vi "temp.vi"   [LabVIEW 2017]
uses:
  Configuration/Controls/Config Data.ctl
  Configuration/Controls/Config CMD.ctl
  ATM Controller/Controls/Controller Overhead.ctl
  ATM Controller/Controls/Controller States.ctl
  ATM Controller/Controls/Controller Message Data.ctl
  ATM Controller/Controls/Controller Message Name.ctl
  Views/User Console View/Controls/User Console - Keypad.ctl
  Views/User Console View/Controls/User Console - Transactions.ctl
  ATM Controller/Controls/Controller CMD.ctl
  Views/User Console View/Controls/User Console - Transaction Enum.ctl
  Error Handler/Controls/Error Data.ctl
  Error Handler/Controls/Error Type.ctl
types:
  T1 = typedef "Controller Message Data.ctl" = cluster{"Transaction":string, "Message":string, "Card Read":bool, "Message Name":T2}
  T2 = typedef "Controller Message Name.ctl" = enum16{"Welcome", "Login", "Idle", "Invalid Login", "Terminate", "Deposit", "Withdrawal", "Fast Cash", "Withdrawal Complete", "Withdrawal Failed", "Balance Inquiry"}
  T3 = typedef "User Console - Transaction Enum.ctl" = enum16{"Balance Inquiry", "Deposit", "Withdrawal", "Fat Cash", "New Transaction", "Terminate Session"}
  T4 = typedef "Controller CMD.ctl" = cluster{"Controller State":T5, "Variant":variant}
  T5 = typedef "Controller States.ctl" = enum16{"Idle", "Init", "Display Message", "Login", "Balance Inquiry", "Deposit", "Withdrawal", "Fast Cash", "Terminate"}
  T6 = typedef "User Console - Transactions.ctl" = cluster{"Balance Inquiry":bool, "Deposit":bool, "Withdrawal":bool, "Fast Cash":bool, "New Transaction":bool, "Terminate":bool}
  T7 = typedef "User Console - Keypad.ctl" = cluster{"Screen":string, "1":bool, "2":bool, "3":bool, "4":bool, "5":bool, "6":bool, "7":bool, "8":bool, "9":bool, "C":bool, "0":bool, "E":bool}
  T8 = typedef "Controller Overhead.ctl" = cluster{"Account found":bool, "Current State":T5, "Next State":T5, "Inactivity Time":dbl, "Account Number":dbl, "Deposit Amount":dbl, "Withdrawal Amount":dbl, "Message Data List":T1[], "Invalid login":i16}
  T9 = typedef "Config CMD.ctl" = enum16{"Read", "Update", "Search"}
  T10 = typedef "Config Data.ctl" = cluster{"Account Number":i32, "Balance":dbl, "First Name":string, "Last Name":string}
  T11 = typedef "Error Data.ctl" = cluster{"Error Type":T12, "Variant":variant}
  T12 = typedef "Error Type.ctl" = enum16{"Console Error", "Sensor Interface IO Error", "Process Step Error"}
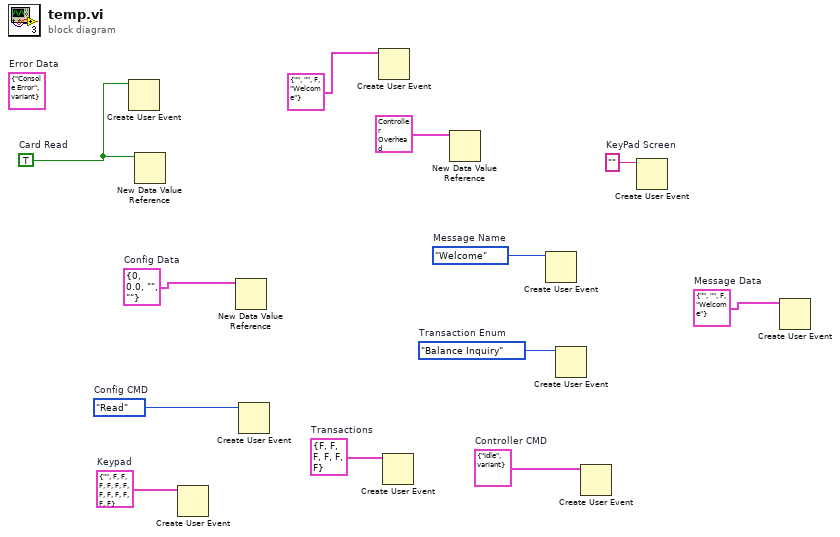
[diagram p0: block diagram]
diagram:
  w1 = T1 {"Transaction"="", "Message"="", "Card Read"=FALSE, "Message Name"=enum."Welcome"}  # Message Data
  w2 = ""  # KeyPad Screen
  w3 = User_Console_-_Transaction_Enum."Balance Inquiry"  # Transaction Enum
  w4 = Controller_Message_Name."Welcome"  # Message Name
  w7 = T4 {"Controller State"=enum."Idle", "Variant"=variant}  # Controller CMD
  w8 = T6 {"Balance Inquiry"=FALSE, "Deposit"=FALSE, "Withdrawal"=FALSE, "Fast Cash"=FALSE, "New Transaction"=FALSE, "Terminate"=FALSE}  # Transactions
  w9 = T7 {"Screen"="", "1"=FALSE, "2"=FALSE, "3"=FALSE, "4"=FALSE, "5"=FALSE, "6"=FALSE, "7"=FALSE, "8"=FALSE, "9"=FALSE, "C"=FALSE, "0"=FALSE, "E"=FALSE}  # Keypad
  w11 = Config_CMD."Read"  # Config CMD
  w5 = T10 {"Account Number"=0, "Balance"=0.0, "First Name"="", "Last Name"=""}  # Config Data
  w12 = TRUE  # Card Read
  (unwired) T11 {"Error Type"=enum."Console Error", "Variant"=variant}  # Error Data
  n1 = Create User Event(user event datatype=w12) -> ()  [unwired: 1 in, 2 out]
  n2 = New Data Value Reference(data value=w12) -> ()  [unwired: 1 in, 2 out]
  n3 = Create User Event(user event datatype=w9) -> ()  [unwired: 1 in, 2 out]
  n4 = New Data Value Reference(data value=w5) -> ()  [unwired: 1 in, 2 out]
  n5 = Create User Event(user event datatype=w11) -> ()  [unwired: 1 in, 2 out]
  n6 = Create User Event(user event datatype=T1 {"Transaction"="", "Message"="", "Card Read"=FALSE, "Message Name"=enum."Welcome"} ("Message Data")) -> ()  [unwired: 1 in, 2 out]
  n7 = Create User Event(user event datatype=w8) -> ()  [unwired: 1 in, 2 out]
  n8 = New Data Value Reference(data value=T8 {"Account found"=FALSE, "Current State"=enum."Idle", "Next State"=enum."Idle", "Inactivity Time"=0.0, "Account Number"=0.0, "Deposit Amount"=0.0, "Withdrawal Amount"=0.0, "Message Data List"=[], "Invalid login"=0} ("Controller Overhead")) -> ()  [unwired: 1 in, 2 out]
  n9 = Create User Event(user event datatype=w4) -> ()  [unwired: 1 in, 2 out]
  n10 = Create User Event(user event datatype=w3) -> ()  [unwired: 1 in, 2 out]
  n11 = Create User Event(user event datatype=w7) -> ()  [unwired: 1 in, 2 out]
  n12 = Create User Event(user event datatype=w2) -> ()  [unwired: 1 in, 2 out]
  n13 = Create User Event(user event datatype=w1) -> ()  [unwired: 1 in, 2 out]
